vi "Setup_CHROMA.vi"() -> (1 "Frequency CHROMA display":dbl, 2 "Voltage CHROMA display":dbl)   [LabVIEW 2013]
uses:
  Global.vi
panel:
  in  "state":u16
  out "error out":errorcluster
  in  "Frequency":dbl(knob) caption="Frequence" min=15.0 max=100.0 step=1.0 scale=15.0..100.0 scale format="%#.0f"
  in  "Voltage":dbl(knob) caption="Tension" min=0.0 max=250.0 step=1.0 scale=0.0..250.0 scale format="%#.1f"
  in  "Preset":u16(ring) items=["Manual Setting", "230 V / 50 Hz", "120 V / 60 Hz", "100 V / 60 Hz"]
  in  "Set setting":bool
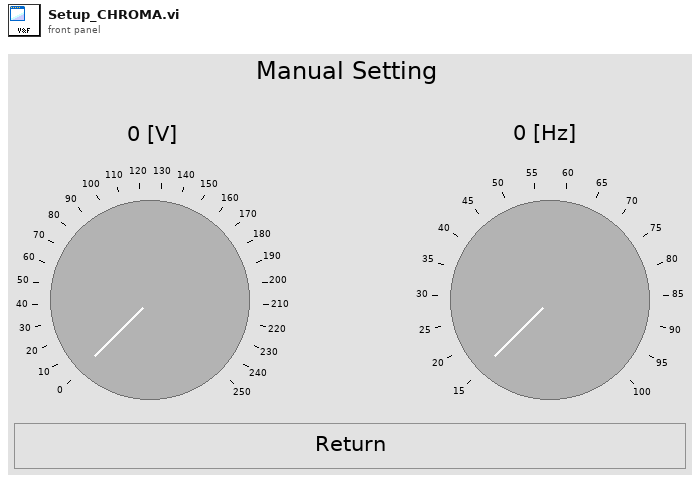
[diagram p1: front panel]
types:
  T1 = enum8{"Enabled", "Disabled", "Disabled and Grayed Out"}
  T2 = cluster{"EMS Status":bool, "Emergency reset":bool, "Voltage CHROMA":sgl, "Frequency CHROMA":sgl, "instrument handle":refnum<k15>, "instrument handle out":refnum<k15>, "virtual keyboard":bool, "Init Procedure":bool}
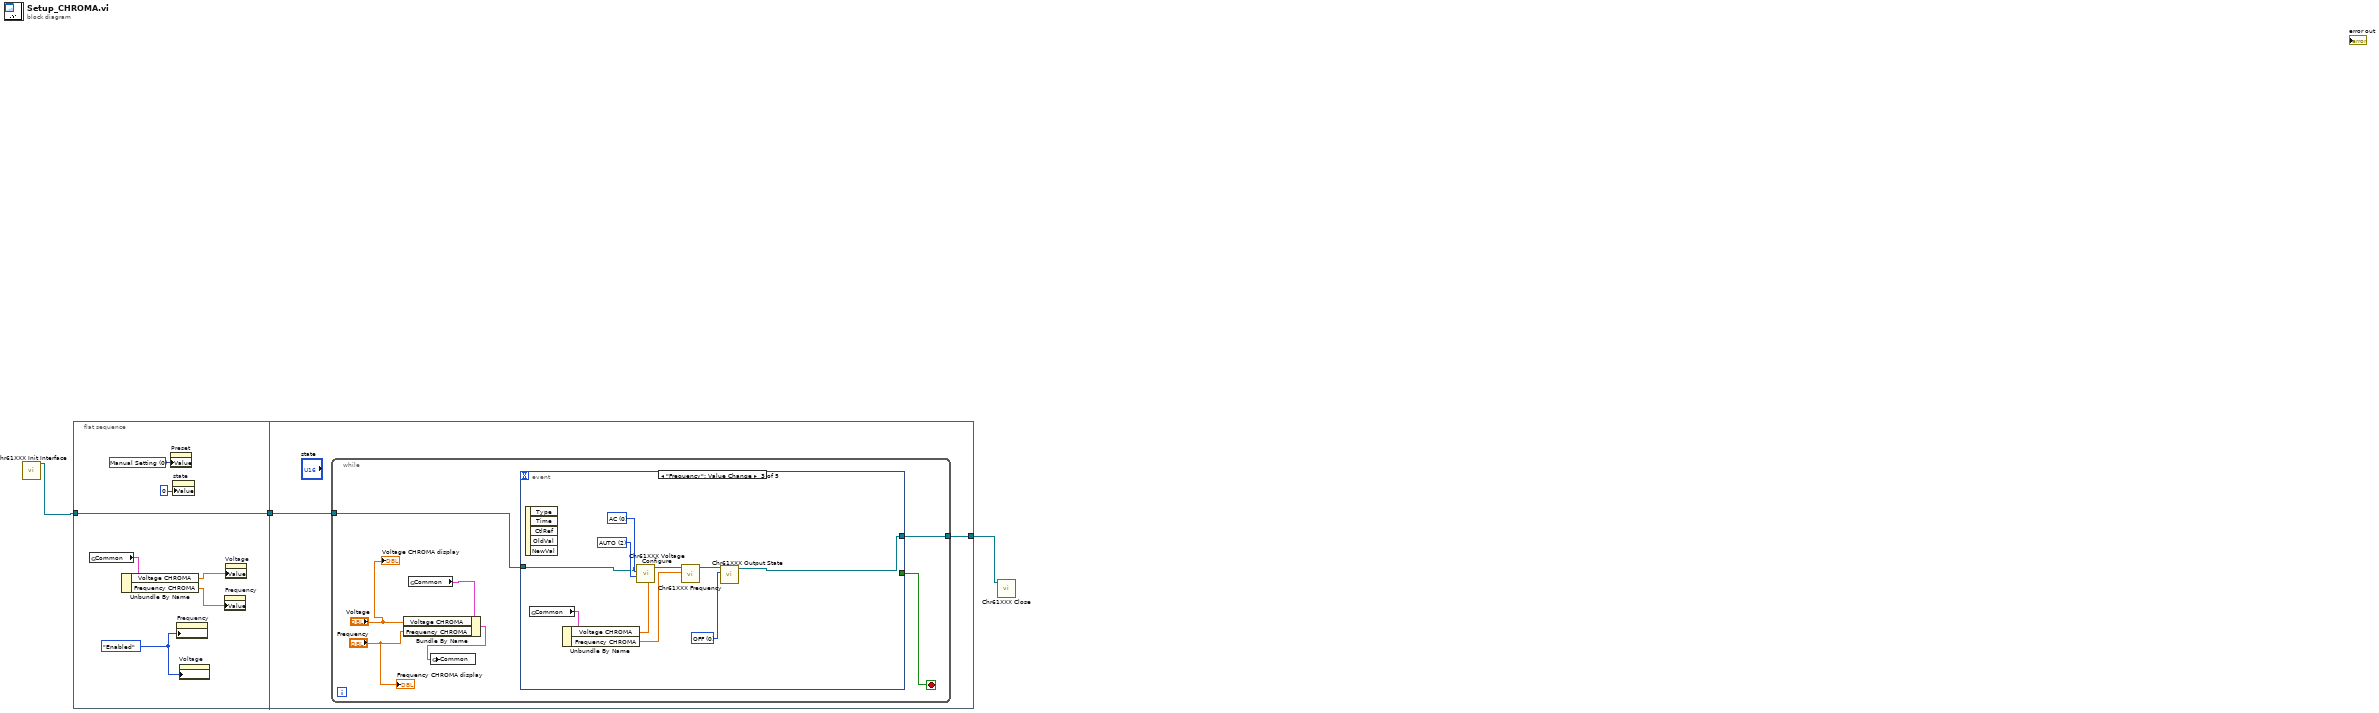
[diagram p0: block diagram]
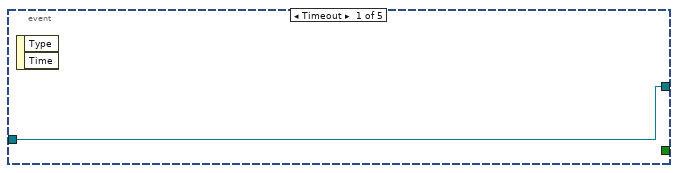
[diagram p2: hidden frame]
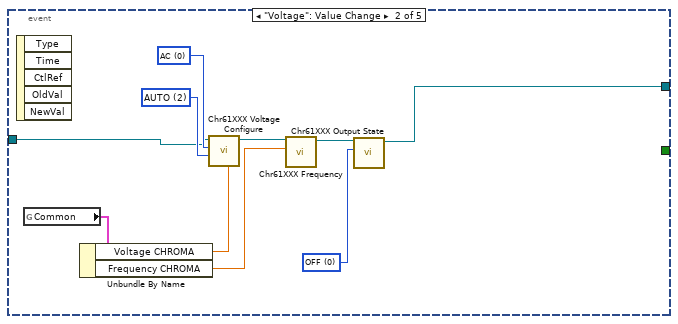
[diagram p3: hidden frame]
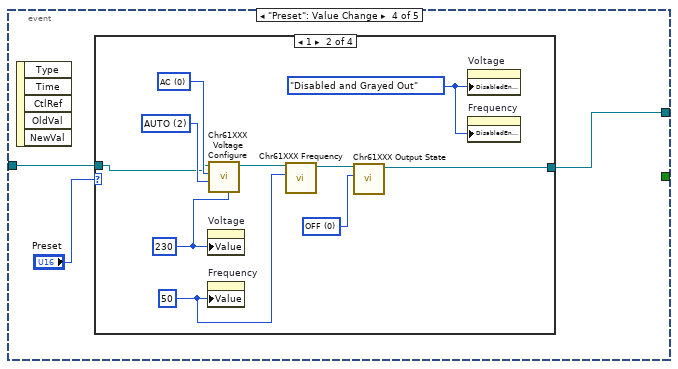
[diagram p4: hidden frame]
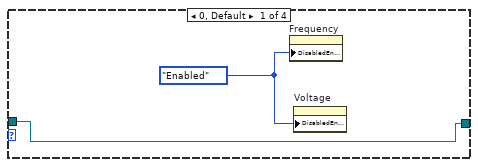
[diagram p5: hidden frame]
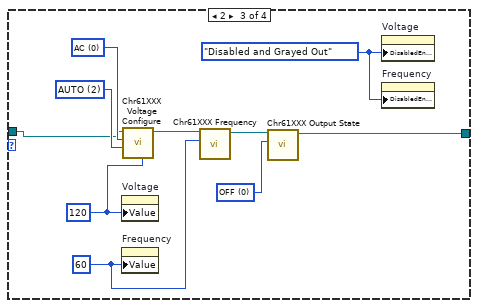
[diagram p6: hidden frame]
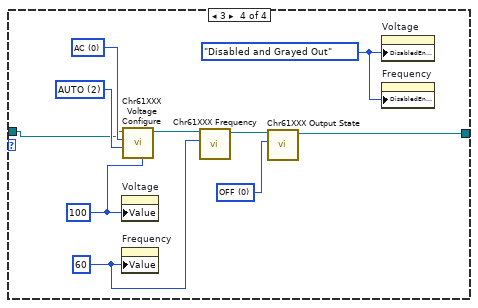
[diagram p7: hidden frame]
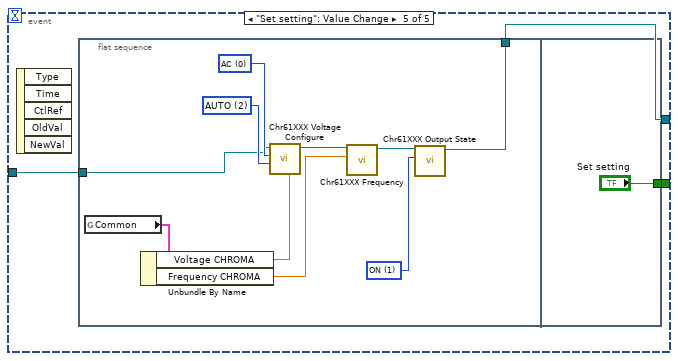
[diagram p8: hidden frame]
diagram:
  n1 = call <instrlib>:"Chr61XXX Init Interface.vi"() -> ("instrument handle out"=w2:refnum<k15>)  [unwired: 9 in, 2 out]
  n2 = flat-sequence {
    tunnel: w2 -> [w10]
    tunnel: [w10] -> w3
    tunnel: [w11] -> w1
    tunnel: w3 -> [w12]
    frame #0 {
      w5 = u16 0 items=["Manual Setting", "230 V / 50 Hz", "120 V / 60 Hz", "100 V / 60 Hz"] ("Preset")
      w6 = T1."Enabled" ("Disabled")
      n3 = global read "Global.vi" "Common"() -> (w9:T2)
      n4 = Unbundle By Name(w9) -> ("Voltage CHROMA"=w8:sgl, "Frequency CHROMA"=w7:sgl)
      n5 = property on="Preset" class="Ring (strict)"("Value"=w5) -> ()  [unwired: 2 in, 2 out]
      n6 = property on="state" class="DigNum (strict)"("Value"=u16 0 ("state")) -> ()  [unwired: 2 in, 2 out]
      n7 = property on="Frequency" class="Knob (strict)"("DisabledEnum"=w6) -> ()  [unwired: 2 in, 2 out]
      n8 = property on="Voltage" class="Knob (strict)"("DisabledEnum"=w6) -> ()  [unwired: 2 in, 2 out]
      n9 = property on="Frequency" class="Knob (strict)"("Value"=w7) -> ()  [unwired: 2 in, 2 out]
      n10 = property on="Voltage" class="Knob (strict)"("Value"=w8) -> ()  [unwired: 2 in, 2 out]
    }
    frame #1 {
      n11 = while {
        tunnel: w12 -> [w14]
        tunnel: [w13] -> w11
        stop <- w17 stop-if-true
        n12 = global read "Global.vi" "Common"() -> (w19:T2)
        n13 = Bundle By Name(cluster=w19, "Voltage CHROMA"="Voltage", "Frequency CHROMA"="Frequency") -> (w18:T2)
        n14 = global write "Global.vi" "Common"(w18) -> ()
        n15 = event shown="[2] \"Frequency\": Value Change" {
          selector: _ -> [_ _ _ _ _]
          dyn-events: _ -> [_ _ _ _ _]
          timeout: _ -> [_ _ _ _ _]
          tunnel: [_ _ _ _ w78] -> w17
          tunnel: w14 -> [w20 w22 w32 w42 w77]
          tunnel: [w20 w21 w31 w41 w76] -> w13
          event Timeout {
            n16 = event-data() -> ()  [unwired: 1 in, 2 out]
          }
          event "Voltage": Value Change {
            w30 = 2 items=["LOW", "HIGH", "AUTO"] ("voltage range")
            w29 = 0 items=["AC", "DC"] ("voltage type")
            w26 = u16 0 items=["OFF", "ON"] ("state")
            n17 = event-data() -> ()  [unwired: 1 in, 5 out]
            n18 = global read "Global.vi" "Common"() -> (w25:T2)
            n19 = Unbundle By Name(w25) -> ("Voltage CHROMA"=w24:sgl, "Frequency CHROMA"=w23:sgl)
            n20 = call <instrlib>:"Chr61XXX Voltage Configure.vi"("voltage"=w24, "voltage range"=w30, "voltage type"=w29, "instrument handle"=w22) -> ("instrument handle out"=w28:refnum<k15>)  [unwired: 6 in, 1 out]
            n21 = call <instrlib>:"Chr61XXX Frequency.vi"("frequency"=w23, "instrument handle"=w28) -> ("instrument handle out"=w27:refnum<k15>)  [unwired: 8 in, 1 out]
            n22 = call <instrlib>:"Chr61XXX Output State.vi"("state"=w26, "instrument handle"=w27) -> ("instrument handle out"=w21:refnum<k15>)  [unwired: 8 in, 1 out]
          }
          event "Frequency": Value Change {
            w40 = 2 items=["LOW", "HIGH", "AUTO"] ("voltage range")
            w39 = 0 items=["AC", "DC"] ("voltage type")
            w36 = u16 0 items=["OFF", "ON"] ("state")
            n23 = event-data() -> ()  [unwired: 1 in, 5 out]
            n24 = global read "Global.vi" "Common"() -> (w35:T2)
            n25 = Unbundle By Name(w35) -> ("Voltage CHROMA"=w34:sgl, "Frequency CHROMA"=w33:sgl)
            n26 = call <instrlib>:"Chr61XXX Voltage Configure.vi"("voltage"=w34, "voltage range"=w40, "voltage type"=w39, "instrument handle"=w32) -> ("instrument handle out"=w38:refnum<k15>)  [unwired: 6 in, 1 out]
            n27 = call <instrlib>:"Chr61XXX Frequency.vi"("frequency"=w33, "instrument handle"=w38) -> ("instrument handle out"=w37:refnum<k15>)  [unwired: 8 in, 1 out]
            n28 = call <instrlib>:"Chr61XXX Output State.vi"("state"=w36, "instrument handle"=w37) -> ("instrument handle out"=w31:refnum<k15>)  [unwired: 8 in, 1 out]
          }
          event "Preset": Value Change {
            n29 = event-data() -> ()  [unwired: 1 in, 5 out]
            n30 = case shown="1" "Preset" {
              tunnel: w42 -> [w44 w46 w56 w67]
              tunnel: [w44 w47 w57 w66] -> w41
              frame 0, Default {
                w45 = T1."Enabled" ("Disabled")
                n31 = property on="Frequency" class="Knob (strict)"("DisabledEnum"=w45) -> ()  [unwired: 2 in, 2 out]
                n32 = property on="Voltage" class="Knob (strict)"("DisabledEnum"=w45) -> ()  [unwired: 2 in, 2 out]
              }
              frame 1 {
                w48 = 50
                w49 = 230
                w50 = T1."Disabled and Grayed Out" ("Disabled")
                w55 = 2 items=["LOW", "HIGH", "AUTO"] ("voltage range")
                w54 = 0 items=["AC", "DC"] ("voltage type")
                w51 = u16 0 items=["OFF", "ON"] ("state")
                n33 = property on="Voltage" class="Knob (strict)"("Value"=w49) -> ()  [unwired: 2 in, 2 out]
                n34 = property on="Frequency" class="Knob (strict)"("Value"=w48) -> ()  [unwired: 2 in, 2 out]
                n35 = call <instrlib>:"Chr61XXX Voltage Configure.vi"("voltage"=w49, "voltage range"=w55, "voltage type"=w54, "instrument handle"=w46) -> ("instrument handle out"=w53:refnum<k15>)  [unwired: 6 in, 1 out]
                n36 = call <instrlib>:"Chr61XXX Frequency.vi"("frequency"=w48, "instrument handle"=w53) -> ("instrument handle out"=w52:refnum<k15>)  [unwired: 8 in, 1 out]
                n37 = call <instrlib>:"Chr61XXX Output State.vi"("state"=w51, "instrument handle"=w52) -> ("instrument handle out"=w47:refnum<k15>)  [unwired: 8 in, 1 out]
                n38 = property on="Voltage" class="Knob (strict)"("DisabledEnum"=w50) -> ()  [unwired: 2 in, 2 out]
                n39 = property on="Frequency" class="Knob (strict)"("DisabledEnum"=w50) -> ()  [unwired: 2 in, 2 out]
              }
              frame 2 {
                w58 = 60
                w59 = 120
                w60 = T1."Disabled and Grayed Out" ("Disabled")
                w65 = 2 items=["LOW", "HIGH", "AUTO"] ("voltage range")
                w64 = 0 items=["AC", "DC"] ("voltage type")
                w61 = u16 0 items=["OFF", "ON"] ("state")
                n40 = property on="Voltage" class="Knob (strict)"("Value"=w59) -> ()  [unwired: 2 in, 2 out]
                n41 = property on="Frequency" class="Knob (strict)"("Value"=w58) -> ()  [unwired: 2 in, 2 out]
                n42 = call <instrlib>:"Chr61XXX Voltage Configure.vi"("voltage"=w59, "voltage range"=w65, "voltage type"=w64, "instrument handle"=w56) -> ("instrument handle out"=w63:refnum<k15>)  [unwired: 6 in, 1 out]
                n43 = call <instrlib>:"Chr61XXX Frequency.vi"("frequency"=w58, "instrument handle"=w63) -> ("instrument handle out"=w62:refnum<k15>)  [unwired: 8 in, 1 out]
                n44 = call <instrlib>:"Chr61XXX Output State.vi"("state"=w61, "instrument handle"=w62) -> ("instrument handle out"=w57:refnum<k15>)  [unwired: 8 in, 1 out]
                n45 = property on="Voltage" class="Knob (strict)"("DisabledEnum"=w60) -> ()  [unwired: 2 in, 2 out]
                n46 = property on="Frequency" class="Knob (strict)"("DisabledEnum"=w60) -> ()  [unwired: 2 in, 2 out]
              }
              frame 3 {
                w68 = 60
                w69 = 100
                w70 = T1."Disabled and Grayed Out" ("Disabled")
                w75 = 2 items=["LOW", "HIGH", "AUTO"] ("voltage range")
                w74 = 0 items=["AC", "DC"] ("voltage type")
                w71 = u16 0 items=["OFF", "ON"] ("state")
                n47 = property on="Voltage" class="Knob (strict)"("Value"=w69) -> ()  [unwired: 2 in, 2 out]
                n48 = property on="Frequency" class="Knob (strict)"("Value"=w68) -> ()  [unwired: 2 in, 2 out]
                n49 = call <instrlib>:"Chr61XXX Voltage Configure.vi"("voltage"=w69, "voltage range"=w75, "voltage type"=w74, "instrument handle"=w67) -> ("instrument handle out"=w73:refnum<k15>)  [unwired: 6 in, 1 out]
                n50 = call <instrlib>:"Chr61XXX Frequency.vi"("frequency"=w68, "instrument handle"=w73) -> ("instrument handle out"=w72:refnum<k15>)  [unwired: 8 in, 1 out]
                n51 = call <instrlib>:"Chr61XXX Output State.vi"("state"=w71, "instrument handle"=w72) -> ("instrument handle out"=w66:refnum<k15>)  [unwired: 8 in, 1 out]
                n52 = property on="Voltage" class="Knob (strict)"("DisabledEnum"=w70) -> ()  [unwired: 2 in, 2 out]
                n53 = property on="Frequency" class="Knob (strict)"("DisabledEnum"=w70) -> ()  [unwired: 2 in, 2 out]
              }
            }
          }
          event "Set setting": Value Change {
            n54 = event-data() -> ()  [unwired: 1 in, 5 out]
            n55 = flat-sequence {
              tunnel: w77 -> [w80]
              tunnel: [w79] -> w76
              tunnel: ["Set setting"] -> w78
              frame #0 {
                w88 = 2 items=["LOW", "HIGH", "AUTO"] ("voltage range")
                w87 = 0 items=["AC", "DC"] ("voltage type")
                w84 = u16 1 items=["OFF", "ON"] ("state")
                n56 = global read "Global.vi" "Common"() -> (w83:T2)
                n57 = Unbundle By Name(w83) -> ("Voltage CHROMA"=w82:sgl, "Frequency CHROMA"=w81:sgl)
                n58 = call <instrlib>:"Chr61XXX Voltage Configure.vi"("voltage"=w82, "voltage range"=w88, "voltage type"=w87, "instrument handle"=w80) -> ("instrument handle out"=w86:refnum<k15>)  [unwired: 6 in, 1 out]
                n59 = call <instrlib>:"Chr61XXX Frequency.vi"("frequency"=w81, "instrument handle"=w86) -> ("instrument handle out"=w85:refnum<k15>)  [unwired: 8 in, 1 out]
                n60 = call <instrlib>:"Chr61XXX Output State.vi"("state"=w84, "instrument handle"=w85) -> ("instrument handle out"=w79:refnum<k15>)  [unwired: 8 in, 1 out]
              }
              frame #1 {
              }
            }
          }
        }
        "Voltage CHROMA display" <- "Voltage"
        "Frequency CHROMA display" <- "Frequency"
      }
    }
  }
  n61 = call <instrlib>:"Chr61XXX Close.vi"("instrument handle"=w1) -> ()  [unwired: 10 in, 1 out]
